vi "Configure Zone.vi"(0 "VISA resource name":refnum<visa-resource-name>, 1 "Manual Heater\nPower (0.000 %)":dbl[](array[numeric]) format="%.3f", 2 "Heater Range (0:Off)":u16[](array[ring]) items=["Off", "Low (loop 1) or On (loop 2)", "High (loop 1)"], 5 "Loop (1:Loop 1)":u16(ring)=1 items=["Loop 1"=1, "Loop 2"=2], 7 "Setpoint\nLimit (0.0000)":dbl[](array[numeric]) format="%.4f", 9 "Gain (P) (0.0)":dbl[](array[numeric]) format="%.1f", 11 "error in (no error)":errorcluster, 12 "Reset (I) (0.0)":dbl[](array[numeric]) format="%.1f", 13 "Rate (D) (0 %)":dbl[](array[numeric])) -> (4 "VISA resource name out":refnum<visa-resource-name>, 6 "Zone":u16[](array[numeric]), 15 "error out":errorcluster)   [LabVIEW 2019, in "Lake Shore 325.lvlib"]
doc: "This VI Configures the parameters of a control loop's zone table. The zone values are configured into arrays to allow all ten zones to be sent each time the vi is executed. The Model 325 allows the user to establish up to 10 custom contiguous temperature zones where the controller will automatically use the pre-programmed PID values and heater ranges. Zone control can be active for both control loops at the same time."
uses:
  Lake Shore 325.lvlib
  Instance           1 22Saved   Configure Zone .vi
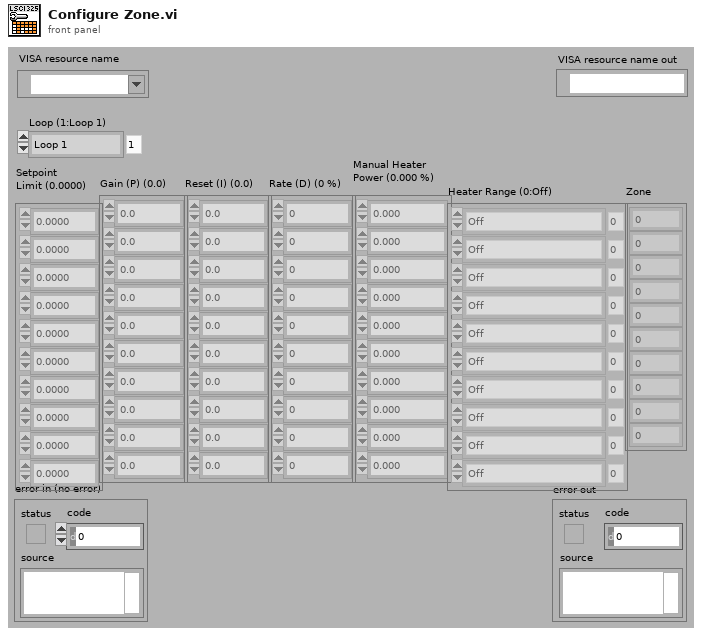
[diagram p1: front panel]
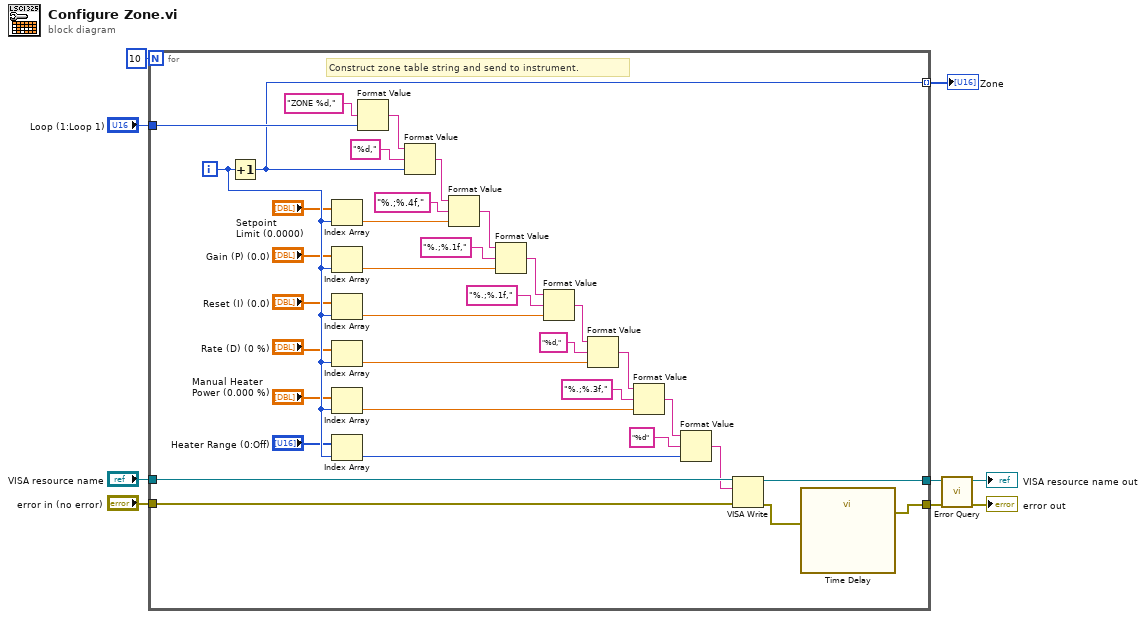
[diagram p0: block diagram]
diagram:
  n1 = for {
    N: 10 -> [_]
    tunnel: "error in (no error)" -> [w44]
    tunnel: "VISA resource name" -> [w45]
    tunnel: [w10] -> w5
    tunnel: [w43] -> w4
    tunnel: "Loop (1:Loop 1)" -> [w28]
    tunnel: [w26] -> w2 mode=indexing
    i -> [w25]
    # "Construct zone table string and send to instrument."
    n2 = Increment(x=w25) -> (x+1=w26:i32)
    n3 = Index Array(array="Setpoint\nLimit (0.0000)", index=w25) -> (element=w18:dbl)
    n4 = Index Array(array="Gain (P) (0.0)", index=w25) -> (element=w17:dbl)
    n5 = Index Array(array="Reset (I) (0.0)", index=w25) -> (element=w16:dbl)
    n6 = Index Array(array="Rate (D) (0 %)", index=w25) -> (element=w15:dbl)
    n7 = Index Array(array="Manual Heater\nPower (0.000 %)", index=w25) -> (element=w14:dbl)
    n8 = Index Array(array="Heater Range (0:Off)", index=w25) -> (element=w13:u16)
    n9 = Format Value(format string="ZONE %d,", value (0)=w28) -> (output string=w33:string)  [unwired: 1 in]
    n10 = Format Value(string ("")=w33, format string="%d,", value (0)=w26) -> (output string=w35:string)
    n11 = Format Value(string ("")=w35, format string="%.;%.4f,", value (0)=w18) -> (output string=w39:string)
    n12 = Format Value(string ("")=w39, format string="%.;%.1f,", value (0)=w17) -> (output string=w40:string)
    n13 = Format Value(string ("")=w40, format string="%.;%.1f,", value (0)=w16) -> (output string=w41:string)
    n14 = Format Value(string ("")=w41, format string="%d,", value (0)=w15) -> (output string=w42:string)
    n15 = Format Value(string ("")=w42, format string="%.;%.3f,", value (0)=w14) -> (output string=w32:string)
    n16 = Format Value(string ("")=w32, format string="%d", value (0)=w13) -> (output string=w12:string)
    n17 = VISA Write(VISA resource name=w45, write buffer=w12, error in (no error)=w44) -> (VISA resource name out=w43:refnum<visa-resource-name>, error out=w11:errorcluster)  [unwired: 1 out]
    n18 = call "Time Delay"("error in (no error)"=w11) -> ("error out"=w10:errorcluster)  [unwired: 10 in]
  }
  "Zone" <- w2
  n19 = call "Error Query.vi"("error in (no error)"=w5, "VISA resource name"=w4) -> ("error out"=→"error out":errorcluster, "VISA resource name out"=→"VISA resource name out":refnum<visa-resource-name>)  [unwired: 7 in, 1 out]
